vi "SetHas Coin State.lvclass.vi"(8 "error in (no error)":errorcluster, 10 "Has Coin State.lvclass":refnum<class "Has Coin State.lvclass">, 11 "reference in":refnum<class "Gum Machine.lvclass">) -> (0 "error out":errorcluster, 3 "reference out":refnum<class "Gum Machine.lvclass">)   [LabVIEW 2013, in "Gum Machine.lvclass"]
uses:
  Gum Machine.lvclass
  Has Coin State_class/Has Coin State.lvclass
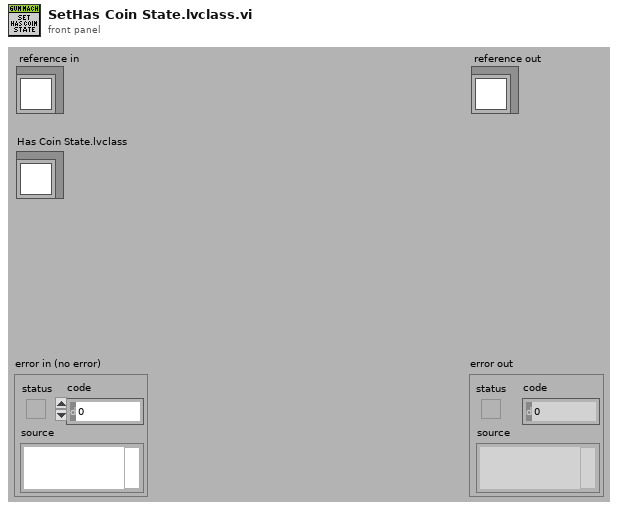
[diagram p1: front panel]
types:
  T1 = typedef "Gum Machine.lvclass/ObjectAttributesRef.ctl" = refnum<data-value>
  T2 = typedef "Gum Machine.lvclass/ObjectAttributes.ctl" = cluster{"No Coin State.lvclass":refnum<class "No Coin State.lvclass">, "Has Coin State.lvclass":refnum<class "Has Coin State.lvclass">, "Sold Out State.lvclass":refnum<class "Sold Out State.lvclass">, "Sold State.lvclass":refnum<class "Sold State.lvclass">, "Number Of Gums":u32, "State.lvclass":refnum<class "State.lvclass">}
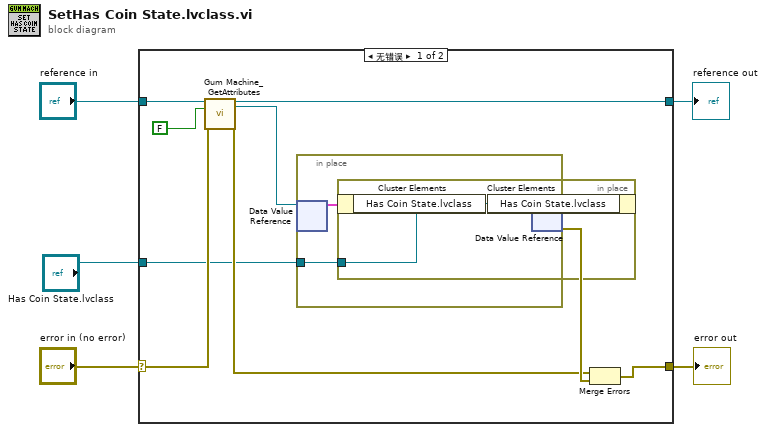
[diagram p0: block diagram]
diagram:
  n1 = case shown="无错误" "error in (no error)" {
    selector: "error in (no error)" -> [w14 w20]
    tunnel: [w8 w20] -> w4
    tunnel: [w13 w19] -> w2
    tunnel: "reference in" -> [w12 w19]
    tunnel: "Has Coin State.lvclass" -> [w6 _]
    frame No Error {
      n2 = call "Gum Machine_GetAttributes.vi"("reference in"=w12, "return data? (T)"=FALSE, "error in (no error)"=w14) -> ("reference out"=w13:refnum<class "Gum Machine.lvclass">, "attributes ref"=w7:T1, "error out"=w9:errorcluster)  [unwired: 13 in, 1 out]
      n3 = in-place {
        in-place-border: w6 -> [w15]
        n4 = in-place-dvr #1(w7) -> (w16:T2)  [unwired: 1 out]
        n5 = in-place {
          in-place-border: w15 -> [w18]
          n6 = in-place-cluster #2(w16) -> ()  [unwired: 1 out]
          n7 = in-place-cluster #2("Has Coin State.lvclass"=w18) -> (w17:T2)
        }
        n8 = in-place-dvr #1(w17) -> (w10:errorcluster)  [unwired: 1 out]
      }
      n9 = Merge Errors(w9, w10) -> (w8:errorcluster)
    }
    frame Error {
    }
  }
  "error out" <- w4
  "reference out" <- w2
